vi "SimpleErrorDialog.vi"(6 "Timeout (-1)":i32=-1, 7 "Blacken (F)":bool, 8 "dialog error":errorcluster) -> (0 "error out":errorcluster, 1 "timed out?":bool)   [LabVIEW 2012]
uses:
  Msg_Error/Msg_Error.lvclass
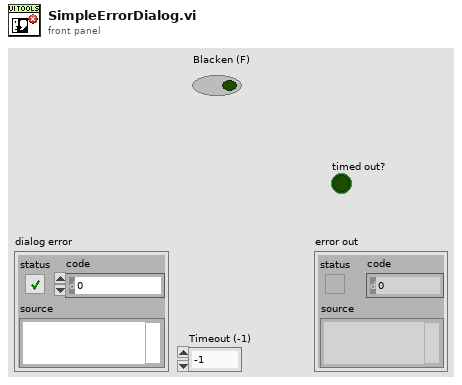
[diagram p1: front panel]
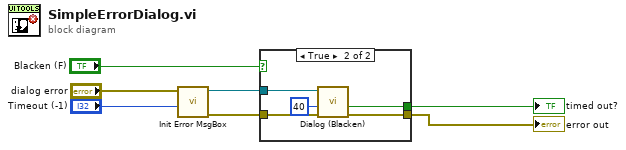
[diagram p0: block diagram]
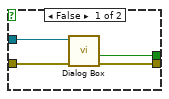
[diagram p2: hidden frame]
diagram:
  n1 = call "Init Error MsgBox.vi"("Timeout (-1)"="Timeout (-1)", "Error"="dialog error") -> ("error out"=w4:errorcluster, "Msg_Error out"=w5:refnum<class "Msg_Error.lvclass">)  [unwired: 8 in]
  n2 = case shown="True" "Blacken (F)" {
    tunnel: w5 -> [w11 w16]
    tunnel: w4 -> [w10 w15]
    tunnel: [w9 w12] -> w3
    tunnel: [w8 w13] -> w2
    frame False {
      n3 = call-dynamic "Dialog Box.vi"("error in (no error)"=w10, "Msg_Error in"=w11) -> ("error out"=w8:errorcluster, "timed out?"=w9:bool)  [unwired: 6 in, 2 out]
    }
    frame True {
      n4 = call-dynamic "Dialog (Blacken).vi"("error in (no error)"=w15, "Transparency (40)"=u8 40, "Dialog in"=w16) -> ("error out"=w13:errorcluster, "timed out?"=w12:bool)  [unwired: 5 in, 2 out]
    }
  }
  "timed out?" <- w3
  "error out" <- w2
